vi "DataLog Save or Load Tag Config.vi"(0 "tag log directory":path, 1 "action":enum16{"save", "load"}(ring), 7 "tag config in":T1 {"logging parameters" format="%.2e"; "precision" items=["0", "1", "2", "3", "4", "5", "6", "7", "8", "9", "10", "11", "12", "13", "14", "15", "16", "17"]; "limit delay" format="%.2e"; "deadband" format="%.2e"}, 11 "error in (no error)":errorcluster) -> (4 "dup tag log directory":path, 8 "tag config out":T1 {"logging parameters" format="%.2e"; "precision" items=["0", "1", "2", "3", "4", "5", "6", "7", "8", "9", "10", "11", "12", "13", "14", "15", "16", "17"]; "limit delay" format="%.2e"; "deadband" format="%.2e"}, 15 "error out":errorcluster)   [LabVIEW 2012]
doc: "Save or load a readable/editable tag configuration file from/to a tag info cluster."
uses:
  typedefs/clusters/t_DataLog Tag Config.ctl
  typedefs/t_DataLog Temporal Types.ctl
  typedefs/t_DataLog Value Types.ctl
  typedefs/t_DataLog Numerical Format.ctl
  typedefs/t_DataLog Logging Algorithms.ctl
  glb_DataLog MCVD.vi
  luaview/subvis/private/LuaVIEW Push (flat data).vi
  luaview/subvis/private/LuaVIEW Pull (string).vi
  luaview/subvis/private/LuaVIEW Push (string).vi
  luaview/subvis/private/LuaVIEW Pull (flat data).vi
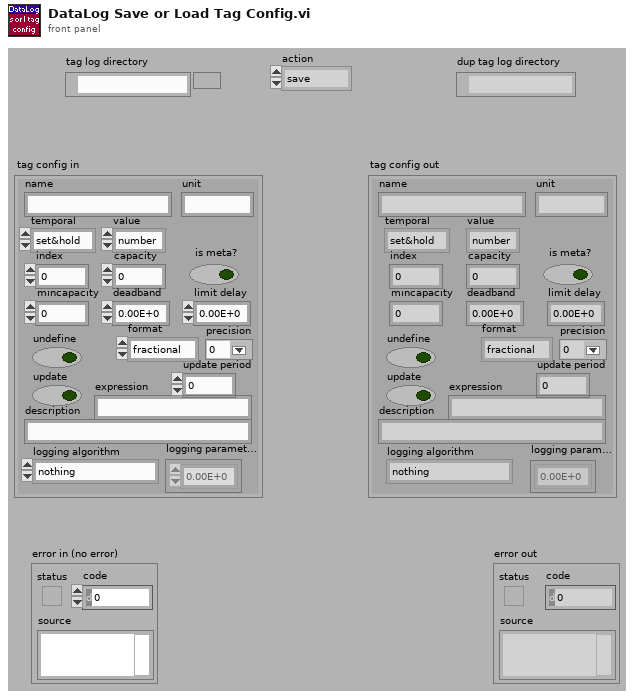
[diagram p1: front panel]
types:
  T1 = typedef "t_DataLog Tag Config.ctl" = cluster{"name":string, "unit":string, "temporal":T2, "value":T3, "index":i32, "capacity":i32, "is meta?":bool, "mincapacity":i32, "deadband":dbl, "limit delay":dbl, "format":T4, "precision":u8, "undefine":bool, "update":bool, "update period":u16, "expression":string, "description":string, "logging algorithm":T5, "logging parameters":dbl[]}
  T2 = typedef "t_DataLog Temporal Types.ctl" = enum16{"set&hold", "sample", "event"}
  T3 = typedef "t_DataLog Value Types.ctl" = enum16{"number", "string"}
  T4 = typedef "t_DataLog Numerical Format.ctl" = enum8{"fractional", "exponential", "engineering"}
  T5 = typedef "t_DataLog Logging Algorithms.ctl" = enum16{"nothing", "changes", "everything", "every Nth", "time threshold", "value threshold + prior", "t or v threshold", "t or v threshold + prior"}
  T6 = typedef "t_LuaVIEW Reference.ctl" = refnum<k1>
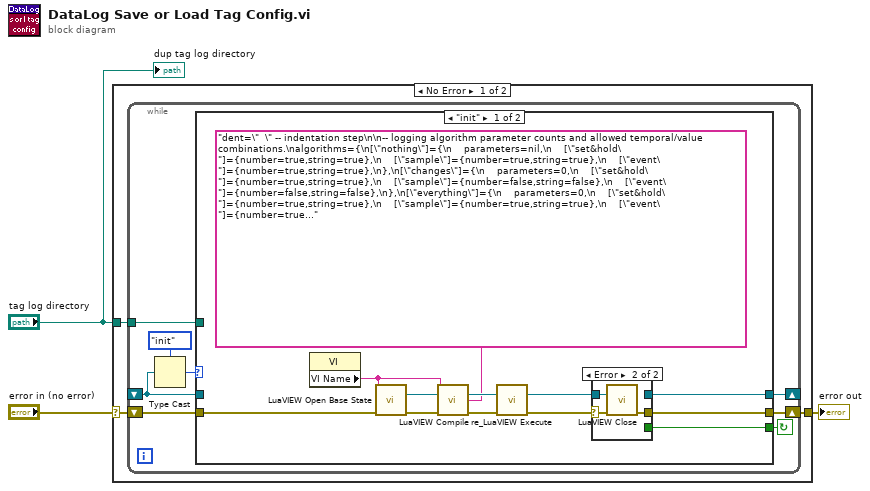
[diagram p0: block diagram]
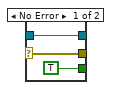
[diagram p2: hidden frame]
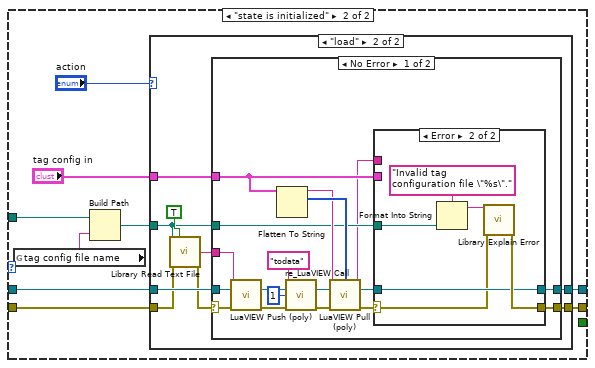
[diagram p3: hidden frame]
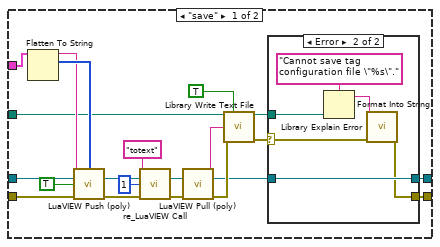
[diagram p4: hidden frame]
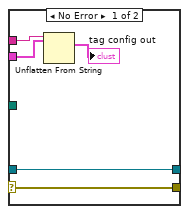
[diagram p6: hidden frame]
diagram:
  n1 = case shown="No Error" "error in (no error)" {
    selector: "error in (no error)" -> [w5 w111]
    tunnel: [w6 w111] -> w2
    tunnel: "tag log directory" -> [w4 _]
    frame No Error {
      n2 = while {
        shift-right: [w13] -> _
        shift-left: _ -> [w11]
        shift-right: [w12] -> w6
        shift-left: w5 -> [w14]
        tunnel: w4 -> [w7]
        stop <- w8 continue-if-true
        n3 = Type Cast(type=enum32{"init", "state is initialized"}."init", x=w11) -> (*(type *) &x=w9:enum32{"init", "state is initialized"})
        n4 = case shown="\"init\"" w9 {
          tunnel: w14 -> [w26 w41]
          tunnel: [w16 w38] -> w13
          tunnel: [w15 w39] -> w12
          tunnel: w11 -> [_ w40]
          tunnel: [w17 _] -> w8
          tunnel: w7 -> [_ w35]
          frame "init" {
            n5 = property class="VI"() -> ("VI Name"=w22:string)  [unwired: 2 in, 2 out]
            n6 = call "LuaVIEW Open Base State.vi"("close identifier (none)"=w22, "error in (no error)"=w26) -> ("LuaVIEW reference"=w24:T6, "error out"=w20:errorcluster)  [unwired: 12 in]
            n7 = call "LuaVIEW Compile.vi"("script name"=w22, "LuaVIEW reference in"=w24, "script"="dent=\"  \" -- indentation step\n\n-- logging algorithm parameter counts and allowed temporal/value combinations.\nalgorithms={\n[\"nothing\"]={\n    parameters=nil,\n    [\"set&hold\"]={number=true,string=true},\n    [\"sample\"]={number=true,string=true},\n    [\"event\"]={number=true,string=true},\n},\n[\"changes\"]={\n    parameters=0,\n    [\"set&hold\"]={number=true,string=true},\n    [\"sample\"]={number=false,string=false},\n    [\"event\"]={number=false,string=false},\n},\n[\"everything\"]={\n    parameters=0,\n    [\"set&hold\"]={number=true,string=true},\n    [\"sample\"]={number=true,string=true},\n    [\"event\"]={number=true,string=true},\n},\n[\"every Nth\"]={\n    parameters=1,\n    [\"set&hold\"]={number=false,string=false},\n    [\"sample\"]={number=true,string=false},\n    [\"event\"]={number=false,string=false},\n    paramcheck=function(params)\n         assert(params[1]>0,\"N parameter should be positive\")\n         assert(params[1]==floor(params[1]),\"N parameter should be an integer\")\n    end\n},\n[\"time threshold\"]={\n    parameters=1,\n    [\"set&hold\"]={number=false,string=false},\n    [\"sample\"]={number=true,string=false},\n    [\"event\"]={number=false,string=false},\n    paramcheck=function(params) assert(params[1]>0,\"time parameter should be positive\") end\n},\n[\"value threshold + prior\"]={\n    parameters=1,\n    [\"set&hold\"]={number=false,string=false},\n    [\"sample\"]={number=true,string=false},\n    [\"event\"]={number=false,string=false},\n    paramcheck=function(params) assert(params[1]>0,\"value parameter should be positive\") end\n},\n[\"t or v threshold\"]={\n    parameters=2,\n    [\"set&hold\"]={number=false,string=false},\n    [\"sample\"]={number=true,string=false},\n    [\"event\"]={number=false,string=false},\n    paramcheck=function(params)\n        assert(params[1]>0,\"time parameter should be positive\")\n        assert(params[2]>0,\"value parameter should be positive\")\n    end\n},\n[\"t or v threshold + prior\"]={\n    parameters=2,\n    [\"set&hold\"]={number=false,string=false},\n    [\"sample\"]={number=true,string=false},\n    [\"event\"]={number=false,string=false},\n    paramcheck=function(params)\n        assert(params[1]>0,\"time parameter should be positive\")\n        assert(params[2]>0,\"value parameter should be positive\")\n    end\n},\n}\n\nfunction arraylike(tab)\n    -- returns a boolean that is true if array like, and the number of keys\n    local keys=0\n    for k,v in pairs(tab) do keys=keys+1 end\n    return table.getn(tab)==keys,keys\nend\n\nfunction check(o)\n    -- check a tag configuration for internal consistency\n    assert(o.value,\"missing value type\")\n    assert(o.temporal,\"missing temporal type\")\n    assert(o.unit,\"missing unit\")\n    assert(o[\"logging algorithm\"],\"no logging algorithm specified\")\n    assert(o[\"logging parameters\"],\"missing logging parameters table\")\n    for i,v in ipairs(o[\"logging parameters\"]) do\n        assert(not lv.isnan(v),\"NaN is not an allowed value for logging parameter #\"..i)\n    end\n    assert(algorithms[o[\"logging algorithm\"]],\"unknown logging algorithm \\\"\"..o[\"logging algorithm\"]..\"\\\" specified\")\n    assert(algorithms[o[\"logging algorithm\"]][o.temporal][o.value],\"logging algorithm \\\"\"..o[\"logging algorithm\"]..\"\\\" is not allowed for tags with \"..o.temporal..\" temporal type and \"..o.value..\" value type\")\n    if algorithms[o[\"logging algorithm\"]][\"parameters\"] then\n        assert(algorithms[o[\"logging algorithm\"]][\"parameters\"]==table.getn(o[\"logging parameters\"]),\"logging algorithm \\\"\"..o[\"logging algorithm\"]..\"\\\" requires precisely \"..algorithms[o[\"logging algorithm\"]][\"parameters\"]..\" parameters.\")\n    end\n    if algorithms[o[\"logging algorithm\"]].paramcheck then\n        algorithms[o[\"logging algorithm\"]].paramcheck(o[\"logging parameters\"])\n    end\n    if o.value==\"string\" then\n        assert(o.unit==\"\",\"string tags must be unitless\")\n        assert(not o.update,\"string tags cannot be updated from an expression\")\n        assert(o.expression==\"\",\"it does not make sense to specify an expression for a string tag\")\n    end\n    if o.update then\n        assert(o.expression~=\"\",\"cannot update an empty expression\")\n        assert(o[\"update period\"]~=0,\"an update period of zero (ms) eats all CPU\")\n    end\n    if o[\"is meta?\"] then\n        assert(o.value==\"number\",\"meta tags must have a number value\")\n        assert(o.temporal==\"set&hold\",\"meta tags must have set&hold temporal type\")\n    end\n    if o.deadband then\n        assert(not lv.isnan(o.deadband),\"NaN is not an allowed value for the dead band\")\n        assert(o.deadband>=0,\"deadband may not be negative\")\n    end\n    if o[\"limit delay\"] then\n        assert(not lv.isnan(o[\"limit delay\"]),\"NaN is not an allowed value for the limit delay\")\n        assert(o[\"limit delay\"]>=0,\"limit delay may not be negative\")\n    end\nend\n\nfunction totext(o)\n    check(o)\n    o.name=nil\n    o.index=nil\n    o.capacity=nil\n    o[\"is meta?\"]=nil\n    return serialize(o,nil,nil)\nend\n\nfunction todata(text)\n    local o=deserialize(text)\n    check(o)\n    return o\nend\n\nfunction serialize(o,indent,incluster)\n    -- pretty format pushed flat data to text (2nd/3rd parameters optional)\n    if not indent then indent=\"\" end\n    local cat={}\n    local typ=type(o)\n    if typ==\"boolean\" then\n        table.insert(cat,tostring(o))\n    elseif typ==\"number\" then\n        if lv.isnan(o) then table.insert(cat,\"_NaN\")\n        elseif lv.isinf(o) then\n            if o>0 then table.insert(cat,\"_Inf\")\n            else table.insert(cat,\"-_Inf\") end\n        else\n            table.insert(cat,tostring(o))\n        end\n    elseif typ==\"string\" then\n        table.insert(cat,string.format(\"%q\",o))\n    elseif typ==\"table\" then\n        local al,keys=arraylike(o)\n        if al and keys == 0 then\n            table.insert(cat,\"{}\")\n        else\n            if incluster then\n                table.insert(cat,\"\\n\"..indent..\"{\\n\")\n            else\n                table.insert(cat,\"{\\n\")\n            end\n            if al then\n                for k,v in ipairs(o) do\n                    table.insert(cat,indent..dent)\n                    table.insert(cat,serialize(v,indent..dent,false))\n                    table.insert(cat,\",\\n\")\n                end\n            else\n                for i,k in ipairs(o._cluster_order) do\n                    if o[k]~=nil then\n                        table.insert(cat,indent..dent..\"[\"..string.format(\"%q\",k)..\"]=\")\n                        table.insert(cat,serialize(o[k],indent..dent,true))\n                        table.insert(cat,\",\\n\")\n                    end\n                end\n            end\n            table.insert(cat,indent..\"}\")\n        end\n    else\n        error(\"cannot serialize a \"..type(o)..\" \")\n    end\n    return table.concat(cat)\nend\n\nfunction deserialize(text)\n    local func,err = loadstring(\"return \"..\"{\"..text..\"}\")\n    if (func) then\n        return func()[1]\n    else\n        error(err)\n    end\nend\n\n-- hide some stuff\nio=nil\nmath=nil\ndebug=nil\n", "error in (no error)"=w20) -> ("LuaVIEW reference out"=w23:T6, "error out"=w25:errorcluster)  [unwired: 10 in]
            n8 = call "re_LuaVIEW Execute.vi"("LuaVIEW reference in"=w23, "error in (no error)"=w25) -> ("LuaVIEW reference out"=w18:T6, "error out"=w19:errorcluster)  [unwired: 12 in]
            n9 = case shown="Error" w19 {
              selector: w19 -> [w28 w32]
              tunnel: w18 -> [w29 w31]
              tunnel: [w28 w30] -> w15
              tunnel: [w29 _] -> w16
              tunnel: [TRUE _] -> w17
              frame No Error {
              }
              frame Error {
                n10 = call "LuaVIEW Close.vi"("LuaVIEW reference"=w31, "error in (no error)"=w32) -> ("dup error"=w30:errorcluster)  [unwired: 13 in]
              }
            }
          }
          frame "state is initialized" {
            n11 = global read "glb_DataLog MCVD.vi" "tag config file name"() -> (w34:string)
            n12 = Build Path(base path=w35, name or relative path=w34) -> (appended path=w33:path)
            n13 = case shown="\"load\"" "action" {
              tunnel: w41 -> [w62 w76]
              tunnel: w40 -> [w61 w77]
              tunnel: [w45 w79] -> w39
              tunnel: [w43 w78] -> w38
              tunnel: "tag config in" -> [w52 w74]
              tunnel: w33 -> [w50 w71]
              frame "save" {
                n14 = Flatten To String(anything=w52) -> (data string=w53:string, type string=w54:i16[])  [unwired: 3 in, 1 out]
                n15 = call-poly "LuaVIEW Push (poly).vi"("flat data"=w53, "type descriptor"=w54, "LuaVIEW reference in"=w61, "include cluster order (false)"=TRUE, "error in (no error)"=w62) -> ("LuaVIEW reference out"=w59:T6, "error out"=w60:errorcluster)  [unwired: 9 in]
                n16 = call "re_LuaVIEW Call.vi"("function name"="totext", "LuaVIEW reference in"=w59, "required results (no checking needed)"=1, "error in (no error)"=w60) -> ("LuaVIEW reference out"=w56:T6, "error out"=w57:errorcluster)  [unwired: 10 in]
                n17 = call-poly "LuaVIEW Pull (poly).vi"("LuaVIEW reference in"=w56, "error in (no error)"=w57) -> ("string"=w51:string, "LuaVIEW reference out"=w44:T6, "error out"=w47:errorcluster)  [unwired: 11 in]
                n18 = call "Library Write Text File.vi"("file path"=w50, "convert eol (F)"=TRUE, "text to write"=w51, "error in (no error)"=w47) -> ("dup path"=w42:path, "error out"=w46:errorcluster)  [unwired: 10 in]
                n19 = case shown="Error" w46 {
                  selector: w46 -> [w63 w66]
                  tunnel: [w63 w65] -> w45
                  tunnel: [w64 w68] -> w43
                  tunnel: w44 -> [w64 w68]
                  tunnel: w42 -> [_ w67]
                  frame No Error {
                  }
                  frame Error {
                    n20 = Format Into String(format string="Cannot save tag configuration file \"%s\".", w67) -> (resulting string=w69:string)  [unwired: 2 in, 1 out]
                    n21 = call "Library Explain Error.vi"("explanation prefix (none)"=w69, "error in (no error)"=w66) -> ("explained error"=w65:errorcluster)  [unwired: 13 in]
                  }
                }
              }
              frame "load" {
                n22 = call "Library Read Text File.vi"("file path"=w71, "convert eol (F)"=TRUE, "error in (no error)"=w76) -> ("read text"=w75:string, "error out"=w72:errorcluster)  [unwired: 10 in, 1 out]
                n23 = case shown="No Error" w72 {
                  selector: w72 -> [w87 w109]
                  tunnel: [w86 w109] -> w79
                  tunnel: [w83 w110] -> w78
                  tunnel: w77 -> [w92 w110]
                  tunnel: w75 -> [w90 _]
                  tunnel: w74 -> [w81 _]
                  tunnel: w71 -> [w85 _]
                  frame No Error {
                    n24 = call-poly "LuaVIEW Push (poly).vi"("string"=w90, "LuaVIEW reference in"=w92, "error in (no error)"=w87) -> ("LuaVIEW reference out"=w96:T6, "error out"=w97:errorcluster)  [unwired: 11 in]
                    n25 = Flatten To String(anything=w81) -> (data string=w89:string, type string=w91:i16[])  [unwired: 3 in, 1 out]
                    n26 = call "re_LuaVIEW Call.vi"("function name"="todata", "LuaVIEW reference in"=w96, "required results (no checking needed)"=1, "error in (no error)"=w97) -> ("LuaVIEW reference out"=w93:T6, "error out"=w94:errorcluster)  [unwired: 10 in]
                    n27 = call-poly "LuaVIEW Pull (poly).vi"("default flat data"=w89, "type descriptor"=w91, "LuaVIEW reference in"=w93, "error in (no error)"=w94) -> ("flat data"=w80:string, "LuaVIEW reference out"=w84:T6, "error out"=w82:errorcluster)  [unwired: 9 in]
                    n28 = case shown="Error" w82 {
                      selector: w82 -> [w101 w103]
                      tunnel: [w101 w106] -> w86
                      tunnel: w85 -> [_ w105]
                      tunnel: w84 -> [w102 w104]
                      tunnel: [w102 w104] -> w83
                      tunnel: w81 -> [w99 _]
                      tunnel: w80 -> [w98 _]
                      frame No Error {
                        n29 = Unflatten From String(type=w99, binary string=w98) -> (value=→"tag config out":T1)  [unwired: 3 in, 2 out]
                      }
                      frame Error {
                        n30 = Format Into String(format string="Invalid tag configuration file \"%s\".", w105) -> (resulting string=w107:string)  [unwired: 2 in, 1 out]
                        n31 = call "Library Explain Error.vi"("explanation prefix (none)"=w107, "error in (no error)"=w103) -> ("explained error"=w106:errorcluster)  [unwired: 13 in]
                      }
                    }
                  }
                  frame Error {
                  }
                }
              }
            }
          }
        }
      }
    }
    frame Error {
    }
  }
  "error out" <- w2
  "dup tag log directory" <- "tag log directory"
